vi "Untitled 1 (SubVI).vi"(4 "Numeric":u8, 6 "Numeric 2":u8, 7 "Numeric 6":u8, 9 "Numeric 3":u8, 10 "Numeric 4":u8, 11 "Numeric 5":u8) -> (3 "String":string)   [LabVIEW 2014]
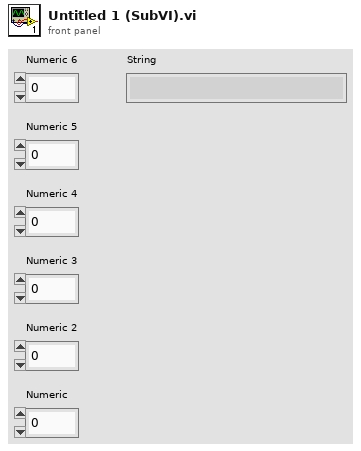
[diagram p1: front panel]
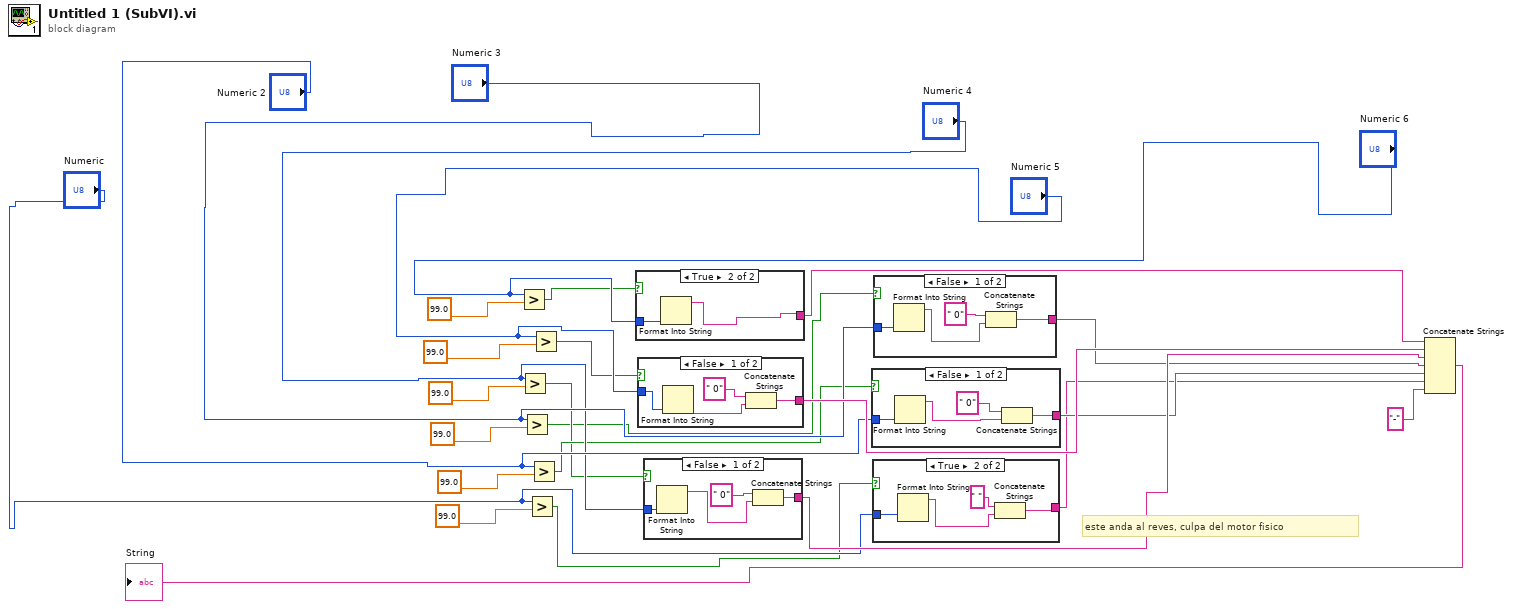
[diagram p0: block diagram]
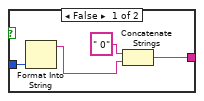
[diagram p2: hidden frame]
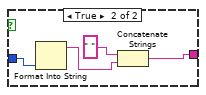
[diagram p3: hidden frame]
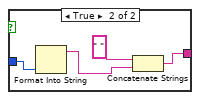
[diagram p4: hidden frame]
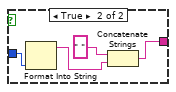
[diagram p5: hidden frame]
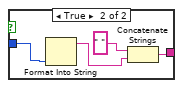
[diagram p6: hidden frame]
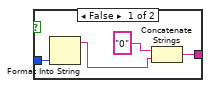
[diagram p7: hidden frame]
diagram:
  # "este anda al reves, culpa del motor fisico"
  n1 = Greater?(x="Numeric 6", y=99.0) -> (0:w9:bool)
  n2 = Greater?(x="Numeric 4", y=99.0) -> (0:w11:bool)
  n3 = Greater?(x="Numeric 3", y=99.0) -> (0:w2:bool)
  n4 = Greater?(x="Numeric", y=99.0) -> (0:w1:bool)
  n5 = Greater?(x="Numeric 2", y=99.0) -> (0:w12:bool)
  n6 = Greater?(x="Numeric 5", y=99.0) -> (0:w10:bool)
  n7 = case shown="True" w9 {
    tunnel: "Numeric 6" -> [w30 w32]
    tunnel: [w27 w31] -> w25
    frame False {
      n8 = Format Into String(w30) -> (resulting string=w28:string)  [unwired: 3 in, 1 out]
      n9 = Concatenate Strings("0" ("string"), w28) -> (w27:string)
    }
    frame True {
      n10 = Format Into String(w32) -> (resulting string=w31:string)  [unwired: 3 in, 1 out]
    }
  }
  n11 = case shown="False" w10 {
    tunnel: "Numeric 5" -> [w34 w37]
    tunnel: [w33 w38] -> w24
    frame False {
      n12 = Format Into String(w34) -> (resulting string=w35:string)  [unwired: 3 in, 1 out]
      n13 = Concatenate Strings(" 0" ("string"), w35) -> (w33:string)
    }
    frame True {
      n14 = Format Into String(w37) -> (resulting string=w39:string)  [unwired: 3 in, 1 out]
      n15 = Concatenate Strings(" " ("string"), w39) -> (w38:string)
    }
  }
  n16 = case shown="False" w11 {
    tunnel: "Numeric 4" -> [w42 w46]
    tunnel: [w41 w45] -> w23
    frame False {
      n17 = Format Into String(w42) -> (resulting string=w43:string)  [unwired: 3 in, 1 out]
      n18 = Concatenate Strings(" 0" ("string"), w43) -> (w41:string)
    }
    frame True {
      n19 = Format Into String(w46) -> (resulting string=w47:string)  [unwired: 3 in, 1 out]
      n20 = Concatenate Strings(" " ("string"), w47) -> (w45:string)
    }
  }
  n21 = case shown="False" w12 {
    tunnel: "Numeric 2" -> [w50 w53]
    tunnel: [w49 w54] -> w21
    frame False {
      n22 = Format Into String(w50) -> (resulting string=w51:string)  [unwired: 3 in, 1 out]
      n23 = Concatenate Strings(" 0" ("string"), w51) -> (w49:string)
    }
    frame True {
      n24 = Format Into String(w53) -> (resulting string=w55:string)  [unwired: 3 in, 1 out]
      n25 = Concatenate Strings(" " ("string"), w55) -> (w54:string)
    }
  }
  n26 = case shown="True" w1 {
    tunnel: "Numeric" -> [w58 w62]
    tunnel: [w57 w61] -> w20
    frame False {
      n27 = Format Into String(w58) -> (resulting string=w59:string)  [unwired: 3 in, 1 out]
      n28 = Concatenate Strings(" 0" ("string"), w59) -> (w57:string)
    }
    frame True {
      n29 = Format Into String(w62) -> (resulting string=w63:string)  [unwired: 3 in, 1 out]
      n30 = Concatenate Strings(" " ("string"), w63) -> (w61:string)
    }
  }
  n31 = case shown="False" w2 {
    tunnel: "Numeric 3" -> [w66 w70]
    tunnel: [w65 w69] -> w22
    frame False {
      n32 = Format Into String(w66) -> (resulting string=w67:string)  [unwired: 3 in, 1 out]
      n33 = Concatenate Strings(" 0" ("string"), w67) -> (w65:string)
    }
    frame True {
      n34 = Format Into String(w70) -> (resulting string=w71:string)  [unwired: 3 in, 1 out]
      n35 = Concatenate Strings(" " ("string"), w71) -> (w69:string)
    }
  }
  n36 = Concatenate Strings(w25, w24, w23, w22, w21, w20, "-" ("string")) -> (→"String":string)
